vi "SMS_GET_OUTPUT.vi"(0 "CRYogenic:(":errorcluster, 1 "Hulk_SMS_addr":refnum<visa-resource-name>) -> (2 "error IO":errorcluster, 3 "read buffer":string, 4 "Numeric":dbl)   [LabVIEW 2021]
uses:
  SMScontrols.ctl
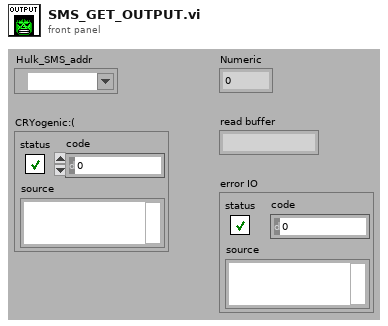
[diagram p1: front panel]
types:
  T1 = typedef "SMScontrols.ctl" = enum16{"UPDATE", "GET OUTPUT", "RAMP ZERO", "RAMP MID", "RAMP MAX", "RAMP STATUS", "PAUSE OFF", "PAUSE ON", "HEATER OFF", "HEATER ON", "TESLA OFF", "TESLA ON", "DIRECTION +", "DIRECTION -", "DIRECTION 0", "SET MID", "SET MAX", "SET RAMP", "SET LIMIT", "SET TPA", "SET HEATER"}
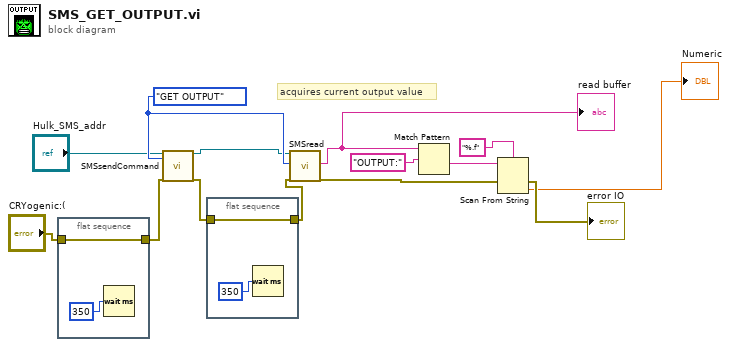
[diagram p0: block diagram]
diagram:
  w7 = SMScontrols."GET OUTPUT" ("SMS controls")
  # "acquires current output value"
  n1 = flat-sequence {
    tunnel: "CRYogenic:(" -> [w15]
    tunnel: [w15] -> w1
    frame #0 {
      n2 = Wait (ms)(milliseconds to wait=u32 350 ("delay[160 ms]")) -> ()  [unwired: 1 out]
    }
  }
  n3 = call "SMSsendCommand.vi"("HULK SMS address in"="Hulk_SMS_addr", "SMS controls"=w7, "error in"=w1) -> ("HULK SMS address out"=w5:refnum<visa-resource-name>, "error out"=w4:errorcluster)  [unwired: 14 in, 1 out]
  n4 = flat-sequence {
    tunnel: w4 -> [w17]
    tunnel: [w17] -> w3
    frame #0 {
      n5 = Wait (ms)(milliseconds to wait=u32 350 ("delay[160 ms]")) -> ()  [unwired: 1 out]
    }
  }
  n6 = call "SMSread.vi"("HULK SMS address in"=w5, "SMS controls"=w7, "error in"=w3) -> ("read buffer"=w12:string, "error out"=w11:errorcluster)  [unwired: 11 in, 4 out]
  "read buffer" <- w12
  n7 = Match Pattern(string=w12, regular expression="OUTPUT:") -> (after substring=w10:string)  [unwired: 1 in, 3 out]
  n8 = Scan From String(format string="%.f", input string=w10, error in=w11) -> (error out=→"error IO":errorcluster, output 1=→"Numeric":dbl)  [unwired: 2 in, 2 out]
